vi "play-AFM-CS-imaging-open-loop.vi"() -> ()   [LabVIEW 2015]
uses:
  raster-scan-params.ctl
  controls/PI-params.ctl
  controls/boolean_info.ctl
  <vilib>/userdefined/High Color/nirio_resource_hc.ctl
  <vilib>/Utility/file.llb/Read Delimited Spreadsheet (DBL).vi
  <vilib>/FPGAPlugInAG/cRIO-9082/niLvFpga_Open_cRIO-9082.vi
  <vilib>/rvi/interface/common/dynamic/niFpgaDynamicAddResources.vi
  <vilib>/FPGAPlugInAG/Dynamic/niLvFpga_Reset_Dynamic.vi
  <vilib>/rvi/interface/common/niFpgaWaitOnOcc.vi
  <vilib>/Utility/error.llb/Error Cluster From Error Code.vi
  <vilib>/rvi/errors/niLvFpgaAdjustHostInterfaceError.vi
  <vilib>/FPGAPlugInAG/Dynamic/niLvFpga_Run_Dynamic.vi
  <vilib>/Utility/file.llb/Write Delimited Spreadsheet (DBL).vi
  <vilib>/FPGAPlugInAG/Dynamic/niLvFpga_Close_Dynamic.vi
  <vilib>/rvi/interface/nirviOpenFPGA/nirviOpenFPGA.xnode
  FPGA Bitfiles/afmimagingcontro_FPGATargetSPARTA_pure-cs-scanning_50aLtqPG5pI.lvbitx
  <vilib>/rvi/interface/nirviMethod/nirviMethod.xnode
  <vilib>/rvi/interface/nirviReadWriteControl/nirviReadWriteControl.xnode
  <vilib>/rvi/interface/nirviCloseFPGA/nirviCloseFPGA.xnode
  <vilib>/FPGAPlugInAG/Dynamic/niLvFpga_ConfigureFifo_Dynamic.vi
  <vilib>/rvi/errors/niLvFpgaMergeErrorWithErrorCode.vi
  <vilib>/rvi/interface/Simulation/niFpgaSimulationCallBeginRW.vi
  <vilib>/FPGAPlugInAG/Dynamic/niLvFpga_ReadFifo_Dynamic.vi
  NiFpgaLv.dll
  <vilib>/FPGAPlugInAG/Dynamic/niLvFpga_WriteFifo_Dynamic.vi
panel:
  in  "zup-N":i16
  out "z-control":dbl[](graph)
  out "x-axis 2":dbl[](graph)
  out "z-error":dbl[](graph)
  out "y-axis 2":dbl[](graph)
  out "size(s) 2":i32[](array[numeric])
  in  "numEntities":i16
  out "uz-":dbl[](graph)
  out "y-axis":dbl[](graph)
  out "x-axis":dbl[](graph)
  in  "z-bound":sgl=5.0
  in  "Ki-xy":sgl=0.005
  out "boolean errors":T1
  in  "raster-scan-params":T2={"TsTicks"=1600, "Stop"=TRUE, "TOL"=0.3, "ramp-rate"=-5e-06, "z-u-max"=5.0, "PI-params"={"Ki"=0.001, "setpoint"=0.0}} {"ramp-rate" format="%#_4g"; "TOL" format="%#_13g"}
  out "e(0) (threshhold init)":fxp<+/-,16,5>
  in  "STOP":bool
  out "nsamps":i32
  in  "trigger-0":bool
  in  "init Z up":sgl
  in  "z_UP (case 3)":sgl=2.0
  out "ADC-zaxis":sgl
  out "elements left":i32=1
  in  "reference traj path":path=path "C:/Users/arnold/Documents/labview/afm_imaging/data/data-in.csv"
  in  "outputData BOTH":path=path "C:/Users/arnold/Documents/labview/afm_imaging/data/data-out.csv"
  out "y iter":i32
  out "size(s)":i32
  in  "x_ffK":dbl=0.307692307692308 format="%#_13g"
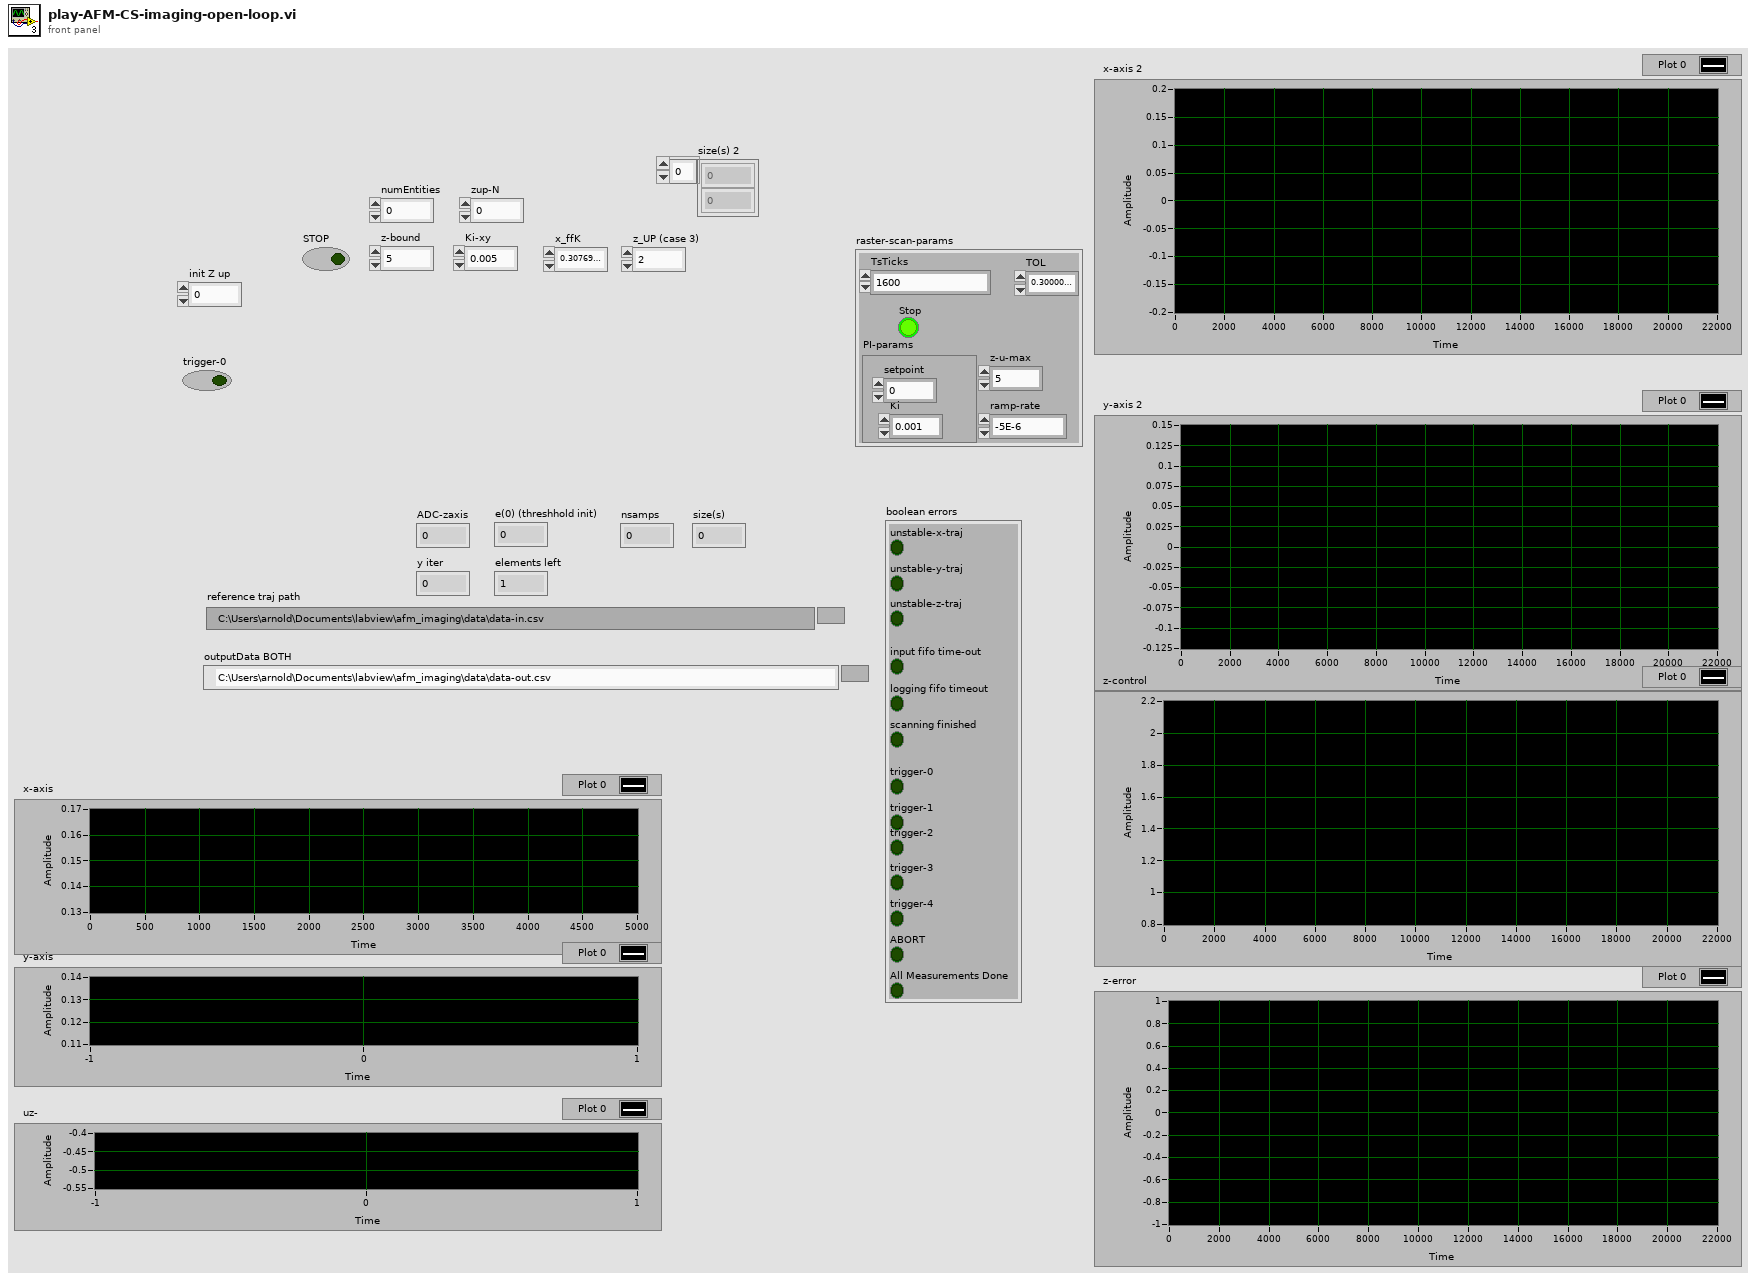
[diagram p1: front panel]
types:
  T1 = typedef "boolean_info.ctl" = cluster{"unstable-z-traj":bool, "input fifo time-out":bool, "logging fifo timeout":bool, "scanning finished":bool, "trigger-1":bool, "trigger-0":bool, "trigger-2":bool, "trigger-3":bool, "trigger-4":bool, "unstable-x-traj":bool, "unstable-y-traj":bool, "ABORT":bool, "All Measurements Done":bool}
  T2 = typedef "raster-scan-params.ctl" = cluster{"TsTicks":u32, "Stop":bool, "TOL":sgl, "ramp-rate":sgl, "z-u-max":sgl, "PI-params":T3}
  T3 = typedef "PI-params.ctl" = cluster{"Ki":sgl, "setpoint":sgl}
  T4 = typedef "nirio_resource_hc.ctl" = tag
  T5 = cluster{"unstable-z-traj":bool, "input fifo time-out":bool, "logging fifo timeout":bool, "scanning finished":bool, "trigger-1":bool, "trigger-0":bool, "trigger-2":bool, "trigger-3":bool, "trigger-4":bool, "unstable-x-traj":bool, "unstable-y-traj":bool, "ABORT":bool, "All Measurements Done":bool}
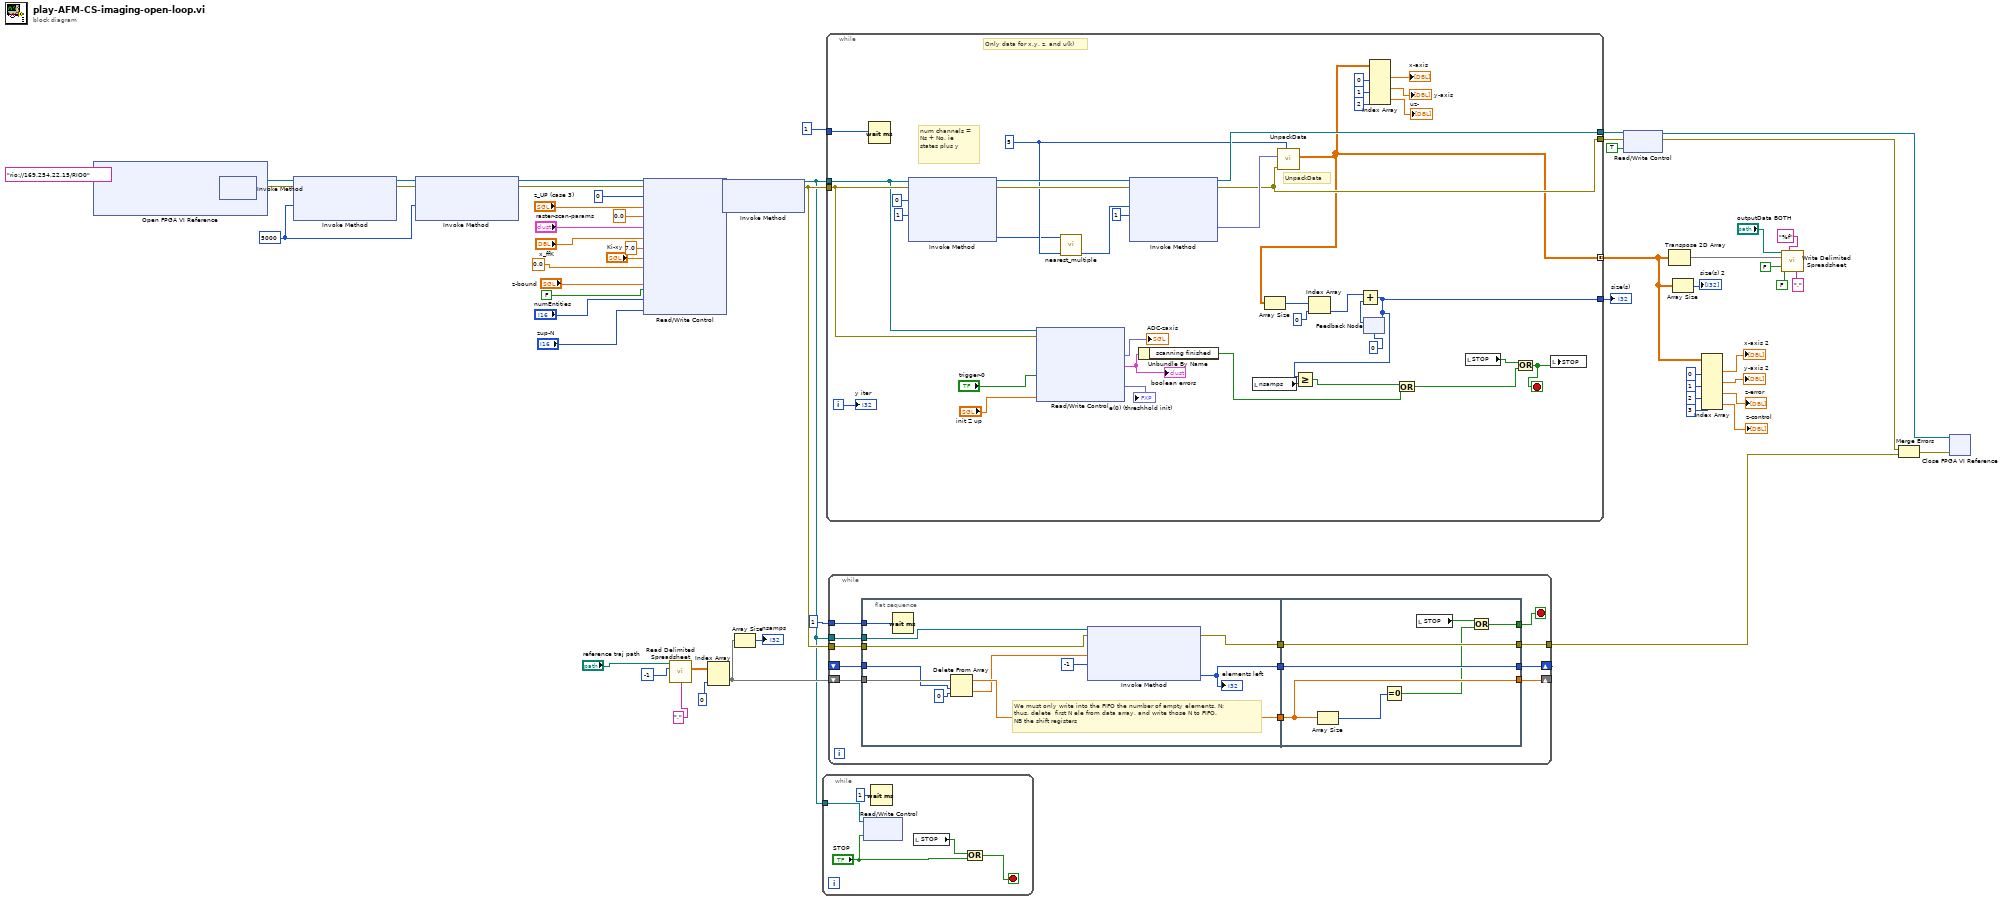
[diagram p0: block diagram]
diagram:
  w55 = 5000
  n1 = xnode "Open FPGA VI Reference"("resource name"=T4 "rio://169.254.22.15/RIO0") -> ("FPGA VI Reference Out"=w54:refnum<k20>, "error out"=w53:errorcluster)  [unwired: 1 in]
  n2 = xnode "Invoke Method"("FPGA VI Reference In"=w54, "error in"=w53) -> ("FPGA VI Reference Out"=w42:refnum<k20>, "error out"=w41:errorcluster)
  n3 = xnode "Invoke Method"("FPGA VI Reference In"=w42, "error in"=w41, "Requested Depth"=w55) -> ("FPGA VI Reference Out"=w46:refnum<k20>, "error out"=w47:errorcluster)  [unwired: 1 out]
  n4 = xnode "Invoke Method"("FPGA VI Reference In"=w46, "error in"=w47, "Requested Depth"=w55) -> ("FPGA VI Reference Out"=w57:refnum<k20>, "error out"=w56:errorcluster)  [unwired: 1 out]
  n5 = xnode "Read/Write Control"("FPGA VI Reference In"=w57, "error in"=w56, "initial case"=i16 0, "z_UP"="z_UP (case 3)", "u_z(0)"=sgl 0.0 ("u(0)"), "raster-scan-params"="raster-scan-params", "x_ffK"="x_ffK", "xy-bound"=sgl 7.0, "Ki-xy"="Ki-xy", "init Z up"=sgl 0.0 ("u(0)"), "z-bound"="z-bound", "trigger-0"=FALSE, "numEntities"="numEntities", "zup-N"="zup-N") -> ("FPGA VI Reference Out"=w44:refnum<k20>, "error out"=w43:errorcluster)
  n6 = call-poly <vilib>:"Read Delimited Spreadsheet.vi"("file path (dialog if empty)"="reference traj path", "number of rows (all:-1)"=-1, "delimiter (\\t)"=",") -> ("all rows"=w31:dbl[][])  [unwired: 7 in, 5 out]
  n7 = Index Array(array=w31, index (col)=0 ("dimension size")) -> (element=w39:dbl[])  [unwired: 1 in]
  n8 = xnode "Invoke Method"("FPGA VI Reference In"=w44, "error in"=w43) -> ("FPGA VI Reference Out"=w1:refnum<k20>, "error out"=w48:errorcluster)  [unwired: 1 in]
  n9 = Array Size(array=w39) -> (size(s)=→"nsamps":i32)
  n10 = while {
    tunnel: w1 -> [w64]
    stop <- w60 stop-if-true
    n11 = xnode "Read/Write Control"("FPGA VI Reference In"=w64, "ABORT"="STOP") -> ()  [unwired: 1 in, 2 out]
    n12 = Wait (ms)(milliseconds to wait=u32 1) -> ()  [unwired: 1 out]
    n13 = local read "STOP"() -> (w61:bool)
    n14 = Or(x=w61, y="STOP") -> (x .or. y?=w60:bool)
  }
  n15 = while {
    tunnel: 1 -> [w103]
    tunnel: w1 -> [w88]
    tunnel: w48 -> [w89]
    tunnel: [w96] -> w24
    tunnel: [w73] -> w5 mode=concatenating
    tunnel: [w86] -> w58
    tunnel: [w74] -> w23
    i -> [w87]
    stop <- w65 stop-if-true
    w79 = u32 5 ("y")
    # "num channels = Ns + No, ie states plus y"
    # "Only data for x,y, z, and u(k)"
    # "UnpackData"
    n16 = Wait (ms)(milliseconds to wait=w103) -> ()  [unwired: 1 out]
    n17 = xnode "Invoke Method"("FPGA VI Reference In"=w88, "error in"=w89, "Number of Elements"=0 ("Timeout (ms)"), "Timeout (ms)"=1) -> ("FPGA VI Reference Out"=w99:refnum<k20>, "error out"=w100:errorcluster, "Elements Remaining"=w78:u32)  [unwired: 1 out]
    n18 = xnode "Read/Write Control"("FPGA VI Reference In"=w88, "error in"=w89, "trigger-0"="trigger-0", "init Z up"="init Z up") -> ("ADC-zaxis"=→"ADC-zaxis":fxp<+/-,24,5>, "boolean indicators"=w76:T5, "e(0) (threshhold init)"=→"e(0) (threshhold init)":fxp<+/-,16,5>)  [unwired: 1 in, 2 out]
    "boolean errors" <- w76
    n19 = call "nearest_multiple.vi"("numChan"=w79, "N"=w78) -> ("(int) y*floor(x/y)"=w77:u64)  [unwired: 9 in]
    n20 = xnode "Invoke Method"("FPGA VI Reference In"=w99, "error in"=w100, "Number of Elements"=w77, "Timeout (ms)"=1) -> ("FPGA VI Reference Out"=w96:refnum<k20>, "error out"=w74:errorcluster, "Data"=w94:fxp<+/-,16,5>[])  [unwired: 1 out]
    n21 = Unbundle By Name(w76) -> ("scanning finished"=w80:bool)
    n22 = local read "nsamps"() -> (w95:i32)
    n23 = call "UnpackData.vi"("NumChannels"=w79, "error In"=w74, "1D Data In"=w94) -> ("2D Data Out"=w73:dbl[][])  [unwired: 7 in, 1 out]
    n24 = Array Size(array=w73) -> (size(s)=w93:i32[])
    n25 = Index Array(array=w93, index=0) -> (element=w91:i32)
    n26 = feedback #1(0) -> (w92:i32)
    n27 = Add(x=w91, y=w92) -> (x+y=w86:i32)
    n28 = Greater Or Equal?(x=w86, y=w95) -> (x >= y?=w75:bool)
    n29 = feedback-in #1(w86) -> ()
    n30 = Index Array(array=w73, index (col) #1=0 ("disabled index (col)"), index (col) #2=1 ("index (col)"), index (col) #3=2 ("index (col)")) -> (element #1=→"x-axis":dbl[], element #2=→"y-axis":dbl[], element #3=→"uz-":dbl[])  [unwired: 3 in]
    n31 = Or(x=w75, y=w80) -> (x .or. y?=w84:bool)
    n32 = local read "STOP"() -> (w66:bool)
    n33 = Or(x=w66, y=w84) -> (x .or. y?=w65:bool)
    n34 = local write "STOP"(w65) -> ()
    "y iter" <- w87
  }
  "size(s)" <- w58
  n35 = while {
    tunnel: [w113] -> w45
    tunnel: 1 -> [w115]
    shift-right: [w109] -> _
    shift-left: _ -> [w112]
    shift-right: [w107] -> _
    shift-left: w39 -> [w114]
    tunnel: w1 -> [w106]
    tunnel: w48 -> [w105]
    stop <- w104 stop-if-true
    n36 = flat-sequence {
      tunnel: w115 -> [w126]
      tunnel: w114 -> [w121]
      tunnel: w112 -> [w117]
      tunnel: [w124] -> w111
      tunnel: [w122] -> w110
      tunnel: [w123] -> w108
      tunnel: w106 -> [w119]
      tunnel: w105 -> [w118]
      tunnel: [w133] -> w109
      tunnel: [w130] -> w113
      tunnel: w111 -> [w130]
      tunnel: w110 -> [w133]
      tunnel: w108 -> [w131]
      tunnel: [w131] -> w107
      tunnel: [w127] -> w104
      frame #0 {
        # "We must only write into the FIFO the number of empty elements, N:\nthus, delete  first N ele from data array, and write those N to FIFO.\nNB the shift registers"
        n37 = Wait (ms)(milliseconds to wait=w126) -> ()  [unwired: 1 out]
        n38 = Delete From Array(array=w121, length=w117, index=0) -> (deleted portion=w120:dbl[], array with subset deleted=w123:dbl[])
        n39 = xnode "Invoke Method"("FPGA VI Reference In"=w119, "error in"=w118, "Data"=w120, "Timeout (ms)"=-1) -> ("error out"=w124:errorcluster, "Empty Elements Remaining"=w122:u32)  [unwired: 1 out]
        "elements left" <- w122
      }
      frame #1 {
        n40 = Array Size(array=w131) -> (size(s)=w132:i32)
        n41 = Equal To 0?(x=w132) -> (x = 0?=w129:bool)
        n42 = local read "STOP"() -> (w128:bool)
        n43 = Or(x=w128, y=w129) -> (x .or. y?=w127:bool)
      }
    }
  }
  n44 = xnode "Read/Write Control"("FPGA VI Reference In"=w24, "error in"=w23, "ABORT"=TRUE) -> ("FPGA VI Reference Out"=w21:refnum<k20>, "error out"=w20:errorcluster)
  n45 = Transpose 2D Array(2D array=w5) -> (transposed array=w28:dbl[][])
  n46 = Array Size(array=w5) -> (size(s)=→"size(s) 2":i32[])
  n47 = Index Array(array=w5, index (col) #1=0 ("disabled index (col)"), index (col) #2=1 ("index (col)"), index (col) #3=2 ("index (col)"), index (col) #4=3 ("index (col)")) -> (element #1=→"x-axis 2":dbl[], element #2=→"y-axis 2":dbl[], element #3=→"z-error":dbl[], element #4=→"z-control":dbl[])  [unwired: 4 in]
  n48 = call-poly <vilib>:"Write Delimited Spreadsheet.vi"("file path (dialog if empty)"="outputData BOTH", "format (%.3f)"="%f", "2D data"=w28, "append to file? (F)"=FALSE, "transpose? (F)"=FALSE, "delimiter (\\t)"=",") -> ()  [unwired: 8 in, 2 out]
  n49 = Merge Errors(w20, w45) -> (w49:errorcluster)
  n50 = xnode "Close FPGA VI Reference"("FPGA VI Reference In"=w21, "error in"=w49) -> ()  [unwired: 1 out]
